vi "build_json.vi"(2 "error in":errorcluster, 4 "Message":string, 5 "Command_ID":string) -> (0 "error out":errorcluster, 1 "JSON Out":string)   [LabVIEW 2025]
doc: "Builds a JSON message to send via TCP with the following format:\n```json\n {\n \"type\": string,\n \"success\": bool,\n \"reference\": int,\n \"message\": JSON\n }\n```"
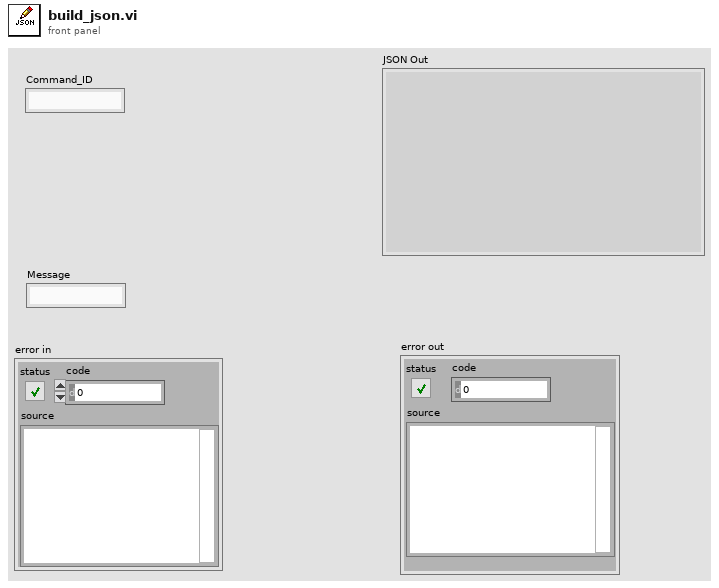
[diagram p1: front panel]
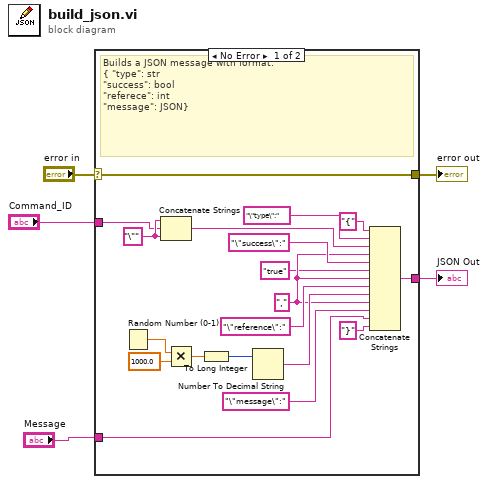
[diagram p0: block diagram]
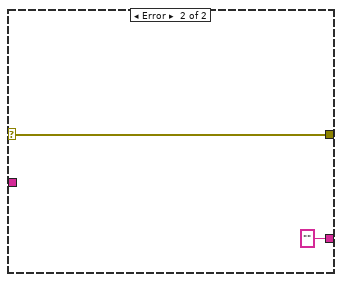
[diagram p2: hidden frame]
diagram:
  n1 = case shown="No Error" "error in" {
    selector: "error in" -> [w14 w26]
    tunnel: [w14 w26] -> w4
    tunnel: "Command_ID" -> [w13 _]
    tunnel: [w12 ""] -> w2
    tunnel: "Message" -> [w6 _]
    frame No Error {
      w19 = "\"" ("string")
      w17 = "," ("string")
      # "Builds a JSON message with format:\n{ \"type\": str\n\"success\": bool\n\"referece\": int\n\"message\": JSON}"
      n2 = Random Number (0-1)() -> (number: 0 to 1=w9:dbl)
      n3 = Concatenate Strings(w19, w13, w19) -> (w18:string)
      n4 = Multiply(x=w9, y=1000.0) -> (x*y=w7:dbl)
      n5 = To Long Integer(number=w7) -> (32bit integer=w11:i32)
      n6 = Number To Decimal String(number=w11) -> (decimal integer string=w20:string)  [unwired: 1 in]
      n7 = Concatenate Strings("{" ("string"), "\"type\":" ("string"), w18, w17, "\"success\":" ("string"), "true" ("string"), w17, "\"reference\":" ("string"), w20, w17, "\"message\":" ("string"), w6, "}" ("string")) -> (w12:string)
    }
    frame Error {
    }
  }
  "error out" <- w4
  "JSON Out" <- w2
